vi "Configure PID Integral Time.vi"(8 "error in (no error)":errorcluster, 10 "integral time, s":dbl=18.0, 11 "HECR in":refnum<class "PL SMC HECR.lvclass">) -> (0 "error out":errorcluster, 3 "HECR out":refnum<class "PL SMC HECR.lvclass">)   [LabVIEW 2015, in "PL SMC HECR.lvclass"]
doc: "Configures PID integral time."
uses:
  PL SMC HECR.lvclass
  <vilib>/plasmapper/PL Modbus Client/PL Modbus Client.lvclass
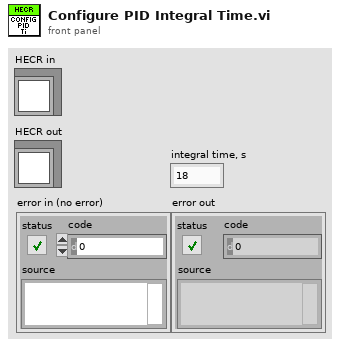
[diagram p1: front panel]
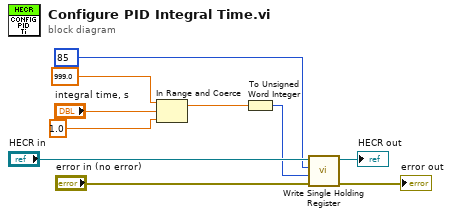
[diagram p0: block diagram]
diagram:
  n1 = In Range and Coerce(upper limit=999.0 ("Ttarget, °C"), x="integral time, s", lower limit=1.0 ("Ttarget, °C")) -> (coerced(x)=w1:dbl)  [unwired: 1 out]
  n2 = To Unsigned Word Integer(number=w1) -> (unsigned 16bit integer=w2:u16)
  n3 = call <vilib>:"Write Single Holding Register.vi"("error in (no error)"="error in (no error)", "value"=w2, "address"=u16 85, "MODBUS in"="HECR in") -> ("error out"=→"error out":errorcluster, "MODBUS out"=→"HECR out":refnum<class "PL SMC HECR.lvclass">)  [unwired: 6 in]
